vi "Setup BC Configuration.vi"(7 "Virtual Memory Unit in":refnum<class "Virtual Memory Unit.lvclass">, 8 "error in (no error)":errorcluster, 11 "Bus Controller in":refnum<class "Bus Controller.lvclass">) -> (0 "error out":errorcluster, 3 "Bus Controller out":refnum<class "Bus Controller.lvclass">, 5 "Virtual Memory Unit out":refnum<class "Virtual Memory Unit.lvclass">)   [LabVIEW 2020, in "BCI-1553 API.lvlib" / "Bus Controller.lvclass"]
doc: "Builds the configuration information for this Bus Contrioller into a single U16 value."
uses:
  Bus Controller.lvclass
  Dependencies/Virtual Memory Unit/Virtual Memory Unit.lvclass
  Bus Controller.lvclass/Bus Controller.ctl
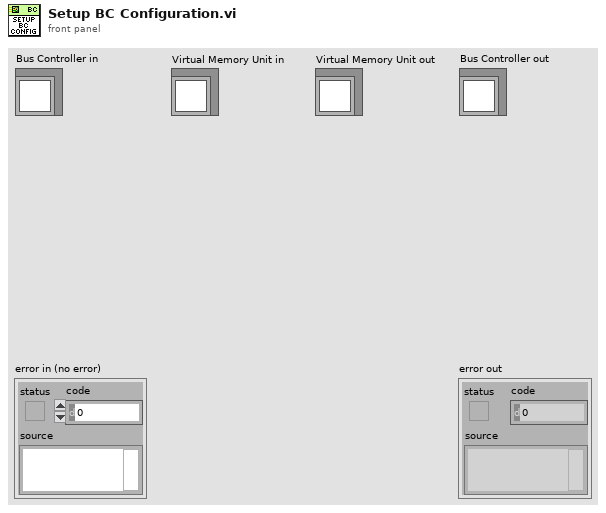
[diagram p1: front panel]
types:
  T1 = typedef "BCI-1553 API.lvlib/Bus Controller.lvclass/Bus Controller Timeout.ctl" = enum16{"17us", "22us", "60us", "140us"}
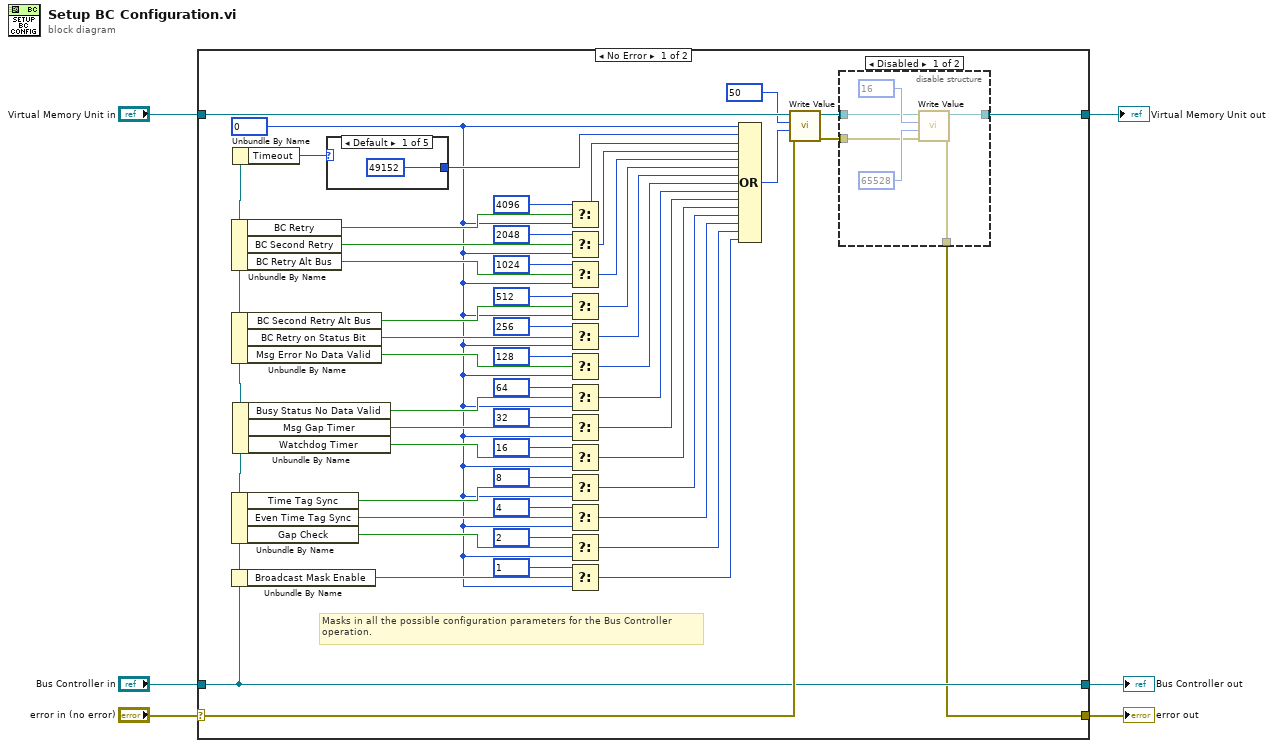
[diagram p0: block diagram]
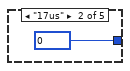
[diagram p3: hidden frame]
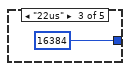
[diagram p4: hidden frame]
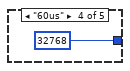
[diagram p5: hidden frame]
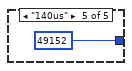
[diagram p6: hidden frame]
diagram:
  n1 = case shown="No Error" "error in (no error)" {
    selector: "error in (no error)" -> [w56 w73]
    tunnel: [w7 w73] -> w2
    tunnel: "Virtual Memory Unit in" -> [w57 w72]
    tunnel: [w9 w72] -> w5
    tunnel: "Bus Controller in" -> [w15 w71]
    tunnel: [w15 w71] -> w3
    frame No Error {
      w12 = u16 0 ("Address")
      # "Masks in all the possible configuration parameters for the Bus Controller\noperation."
      n2 = Unbundle By Name(w15) -> ("BC Retry"=w50:bool, "BC Second Retry"=w47:bool, "BC Retry Alt Bus"=w46:bool)
      n3 = Unbundle By Name(w15) -> ("BC Second Retry Alt Bus"=w37:bool, "BC Retry on Status Bit"=w39:bool, "Msg Error No Data Valid"=w38:bool)
      n4 = Unbundle By Name(w15) -> ("Time Tag Sync"=w20:bool, "Even Time Tag Sync"=w21:bool, "Gap Check"=w19:bool)
      n5 = Unbundle By Name(w15) -> ("Broadcast Mask Enable"=w13:bool)
      n6 = Unbundle By Name(w15) -> ("Timeout"=w53:T1)
      n7 = Unbundle By Name(w15) -> ("Busy Status No Data Valid"=w31:bool, "Msg Gap Timer"=w32:bool, "Watchdog Timer"=w30:bool)
      n8 = case shown="Default" w53 {
        tunnel: [u16 49152 ("Address") u16 0 ("Address") u16 16384 ("Address") u16 32768 ("Address") u16 49152 ("Address")] -> w52
        frame Default {
        }
        frame "17us" {
        }
        frame "22us" {
        }
        frame "60us" {
        }
        frame "140us" {
        }
      }
      n9 = Select(t=u16 4096 ("Address"), s=w50, f=w12) -> (s? t:f=w45:u16)
      n10 = Select(t=u16 2048 ("Address"), s=w47, f=w12) -> (s? t:f=w44:u16)
      n11 = Select(t=u16 1024 ("Address"), s=w46, f=w12) -> (s? t:f=w43:u16)
      n12 = Select(t=u16 512 ("Address"), s=w37, f=w12) -> (s? t:f=w36:u16)
      n13 = Select(t=u16 256 ("Address"), s=w39, f=w12) -> (s? t:f=w35:u16)
      n14 = Select(t=u16 128 ("Address"), s=w38, f=w12) -> (s? t:f=w28:u16)
      n15 = Select(t=u16 64 ("Address"), s=w31, f=w12) -> (s? t:f=w27:u16)
      n16 = Select(t=u16 32 ("Address"), s=w32, f=w12) -> (s? t:f=w26:u16)
      n17 = Select(t=u16 16 ("Address"), s=w30, f=w12) -> (s? t:f=w25:u16)
      n18 = Select(t=u16 8 ("Address"), s=w20, f=w12) -> (s? t:f=w18:u16)
      n19 = Select(t=u16 4 ("Address"), s=w21, f=w12) -> (s? t:f=w17:u16)
      n20 = Select(t=u16 2 ("Address"), s=w19, f=w12) -> (s? t:f=w16:u16)
      n21 = Select(t=u16 1 ("Address"), s=w13, f=w12) -> (s? t:f=w11:u16)
      n22 = Compound Arithmetic op=OR(w12, w52, w45, w44, w43, w36, w35, w28, w27, w26, w25, w18, w17, w16, w11) -> (w54:u16)
      n23 = call "Write Value.vi"("error in (no error)"=w56, "Value"=w54, "Index"=50 ("Address"), "Virtual Memory Unit in"=w57) -> ("error out"=w8:errorcluster, "Virtual Memory Unit out"=w10:refnum<class "Virtual Memory Unit.lvclass">)  [unwired: 6 in]
      n24 = disable-structure shown="Disabled" {
        disable-tunnel: w10 -> [w62 w65]
        disable-tunnel: [w61 w65] -> w9
        disable-tunnel: w8 -> [w59 w64]
        disable-tunnel: [w58 w64] -> w7
        frame Disabled {
          n25 = call "Write Value.vi"("error in (no error)"=w59, "Value"=u16 65528 ("Address"), "Index"=16 ("Address"), "Virtual Memory Unit in"=w62) -> ("error out"=w58:errorcluster, "Virtual Memory Unit out"=w61:refnum<class "Virtual Memory Unit.lvclass">)  [unwired: 6 in]
        }
        frame Enabled {
        }
      }
    }
    frame Error {
    }
  }
  "error out" <- w2
  "Bus Controller out" <- w3
  "Virtual Memory Unit out" <- w5
